vi "Autonomous Independent.vi"   [LabVIEW 2017]
doc: "This VI is called when autonomous begins, and will automatically be terminated when autonomous ends. You can carry out timed or sensor driven robot movement independently without needing to return to the caller."
uses:
  <vilib>/Rock Robotics/WPI/Utilities/WPI_GetSetVariantRefNum.vi
  <vilib>/Rock Robotics/Network Tables/NT Read String.vi
  <vilib>/Rock Robotics/Network Tables/NT Write Numeric Array.vi
  <vilib>/Rock Robotics/Network Tables/NT Read Number.vi
  <vilib>/Rock Robotics/Network Tables/NT Read Boolean.vi
panel:
  # "Be sure to right-click and choose Data Operations>>Make Current Value default if you want to save the array values with the VI"
types:
  T1 = typedef "WPI_JoystickDevRef.ctl" = cluster{"Device":T2}
  T2 = typedef "WPI_JoystickDeviceEnum.ctl" = enum16{"USB 0", "USB 1", "USB 2", "USB 3", "USB 4", "USB 5"}
  T3 = typedef "WPI_RobotDriveDevRef.ctl" = cluster{"DevStatus":errorcluster, "Motors[]":T4[], "Square Inputs":bool, "Max Output":dbl}
  T4 = typedef "WPI_MotorControlDeviceRef.ctl" = cluster{"DeviceStatus":errorcluster, "Type":T5, "PWM":cluster{"PWM Channel":T6, "DeadBand":T7}, "CAN":cluster{"Device Number":u8, "SetOutput VI Ref":variant, "GetOutput VI Ref":variant, "Enable VI Ref":variant, "Disable VI Ref":variant, "Data":variant}, "Invert":bool, "DIO PWM":cluster{"PWM \"Enable\" Channel":T6, "DIOChannel":T8, "PWM Rate":dbl}}
  T5 = typedef "WPI_MotorControlType.ctl" = enum16{"PWM", "CAN", "DIO PWM"}
  T6 = typedef "FPGA_DIOPWMChannel.ctl" = enum8{"PWM 0", "PWM 1", "PWM 2", "PWM 3", "PWM 4", "PWM 5", "PWM 6", "PWM 7", "PWM 8", "PWM 9", "PWM MXP 0", "PWM MXP 1", "PWM MXP 2", "PWM MXP 3", "PWM MXP 4", "PWM MXP 5", "PWM MXP 6", "PWM MXP 7", "PWM MXP 8", "PWM MXP 9", "Invalid"}
  T7 = typedef "WPI_PWMDeadband.ctl" = cluster{"Name":string, "maxPositivePwm":i32, "minPositivePwm":i32, "centerPwm":i32, "maxNegativePwm":i32, "minNegativePwm":i32, "angularRange":u16}
  T8 = typedef "FPGA_DIOChannel.ctl" = enum8{"DIO 0", "DIO 1", "DIO 2", "DIO 3", "DIO 4", "DIO 5", "DIO 6", "DIO 7", "DIO 8", "DIO 9", "DIO MXP 0", "DIO MXP 1", "DIO MXP 2", "DIO MXP 3", "DIO MXP 4", "DIO MXP 5", "DIO MXP 6", "DIO MXP 7", "DIO MXP 8", "DIO MXP 9", "DIO MXP 10", "DIO MXP 11", "DIO MXP 12", "DIO MXP 13", "DIO MXP 14", "DIO MXP 15", "SPI Port CS1", "SPI Port CS2", "SPI Port CS3", "SPI Port MISO", "SPI Port MOSI", "Invalid"}
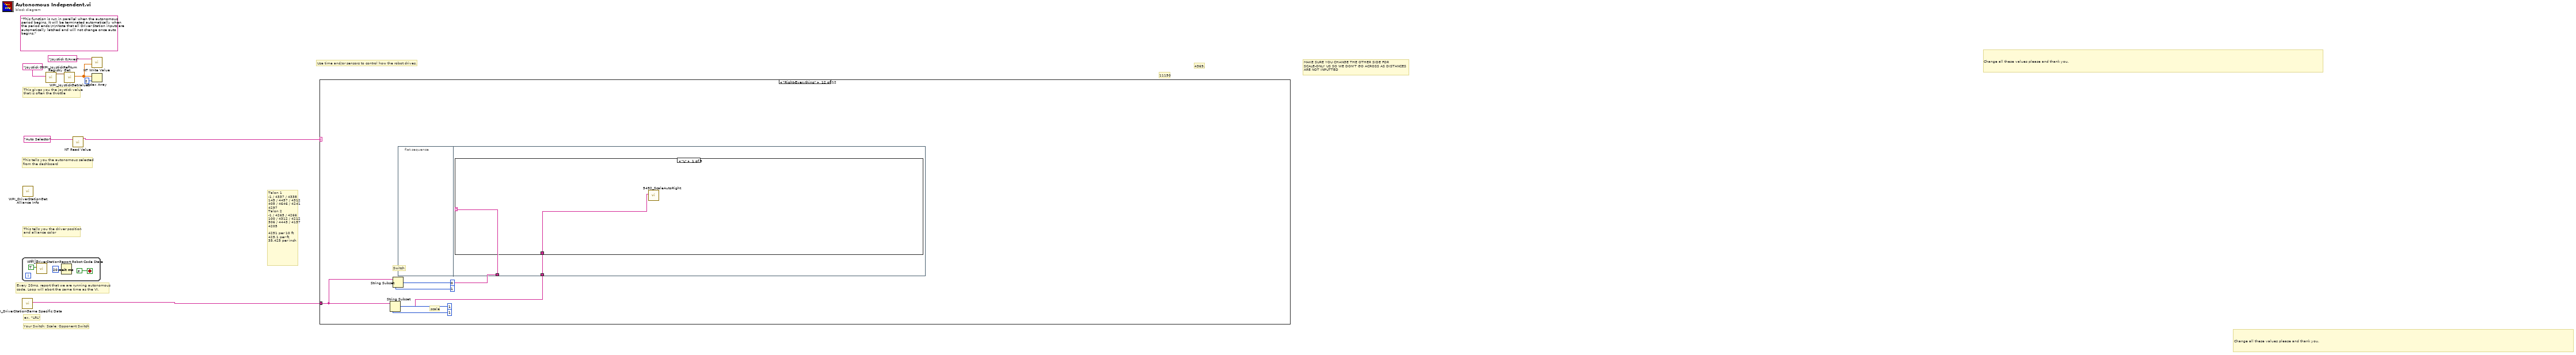
[diagram p0: block diagram]
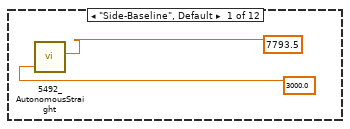
[diagram p2: hidden frame]
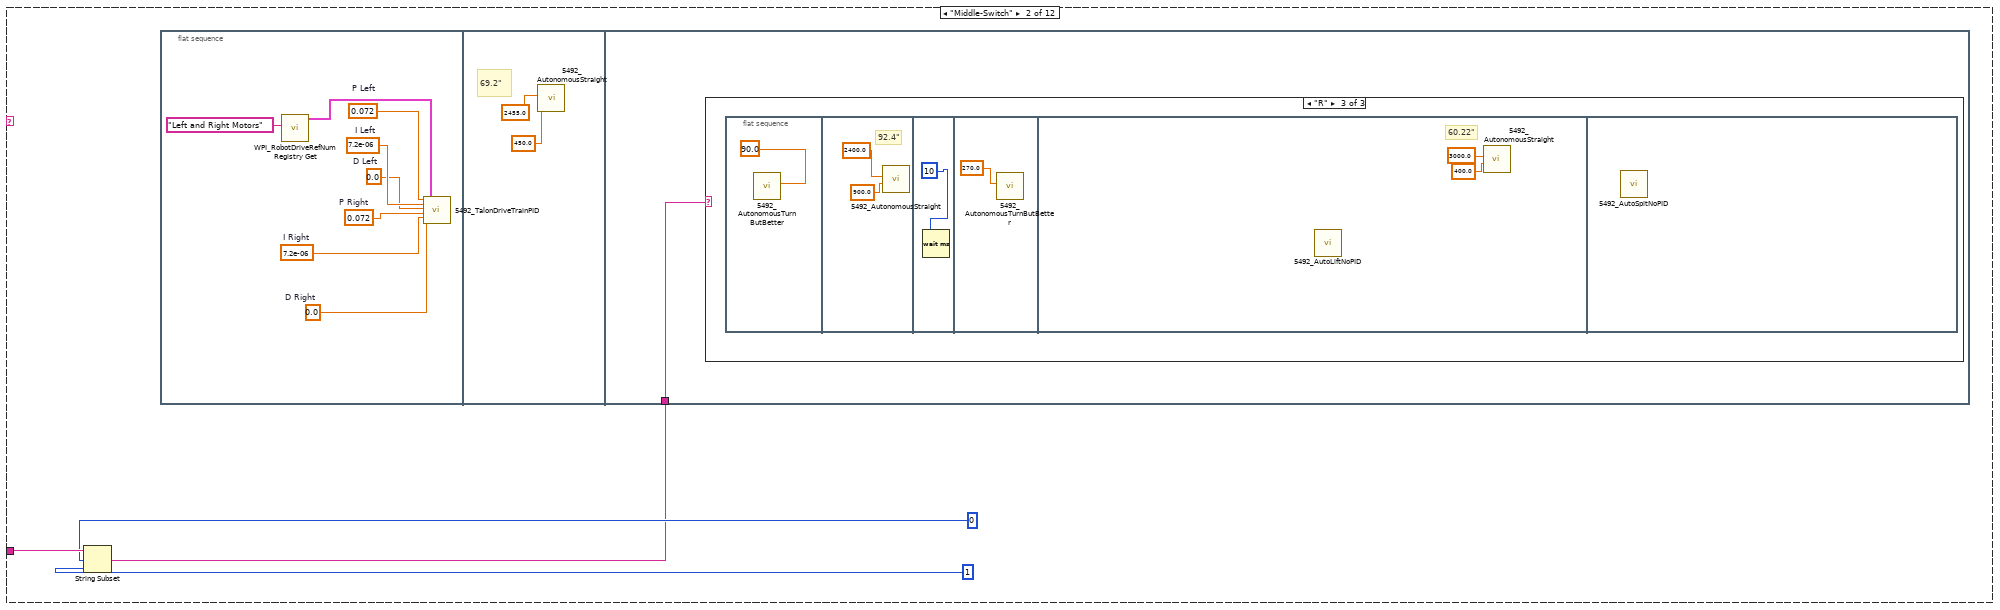
[diagram p3: hidden frame]
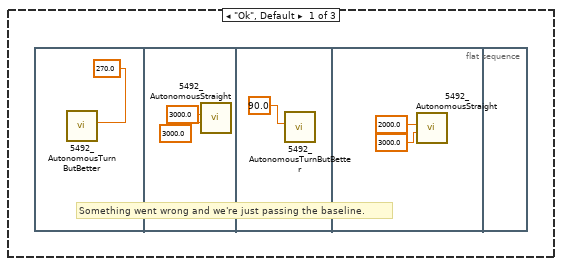
[diagram p4: hidden frame]
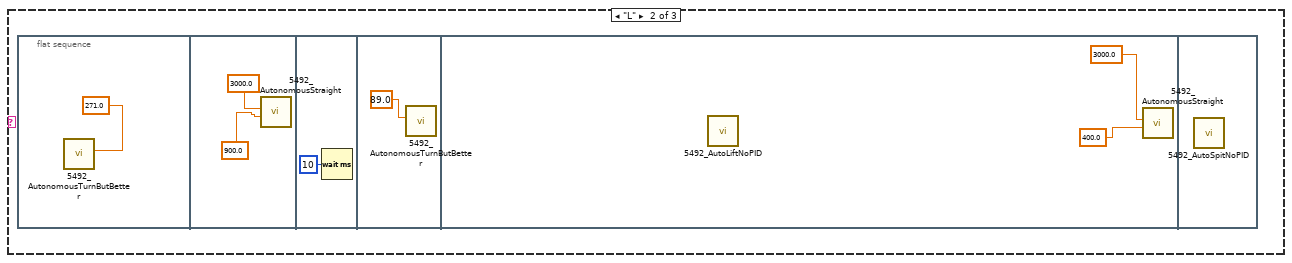
[diagram p5: hidden frame]
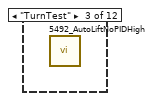
[diagram p6: hidden frame]
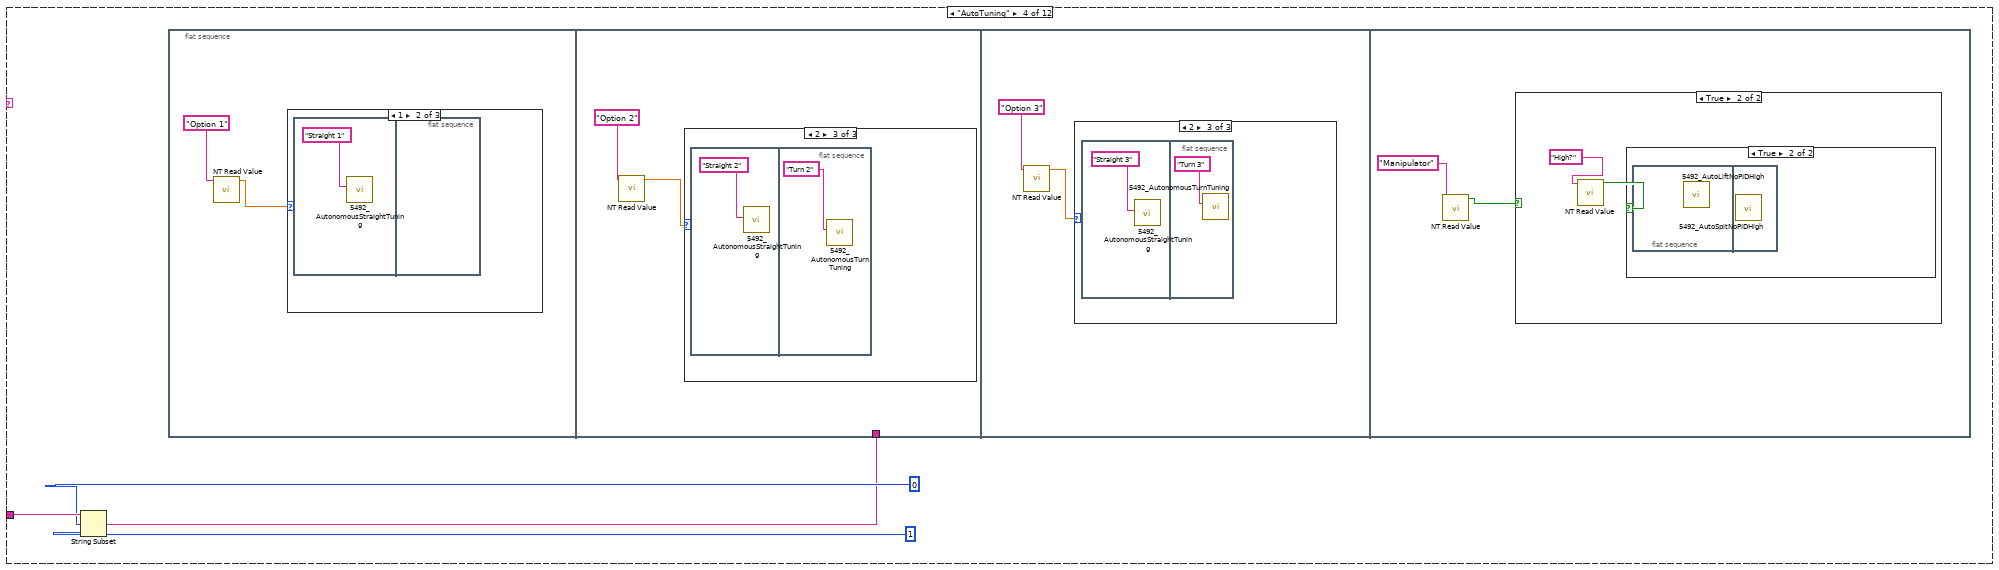
[diagram p7: hidden frame]
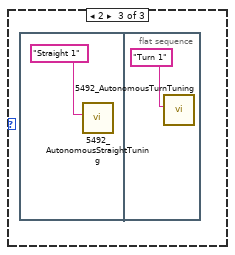
[diagram p9: hidden frame]
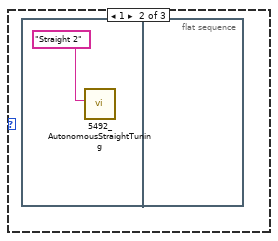
[diagram p11: hidden frame]
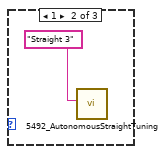
[diagram p13: hidden frame]
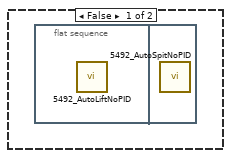
[diagram p15: hidden frame]
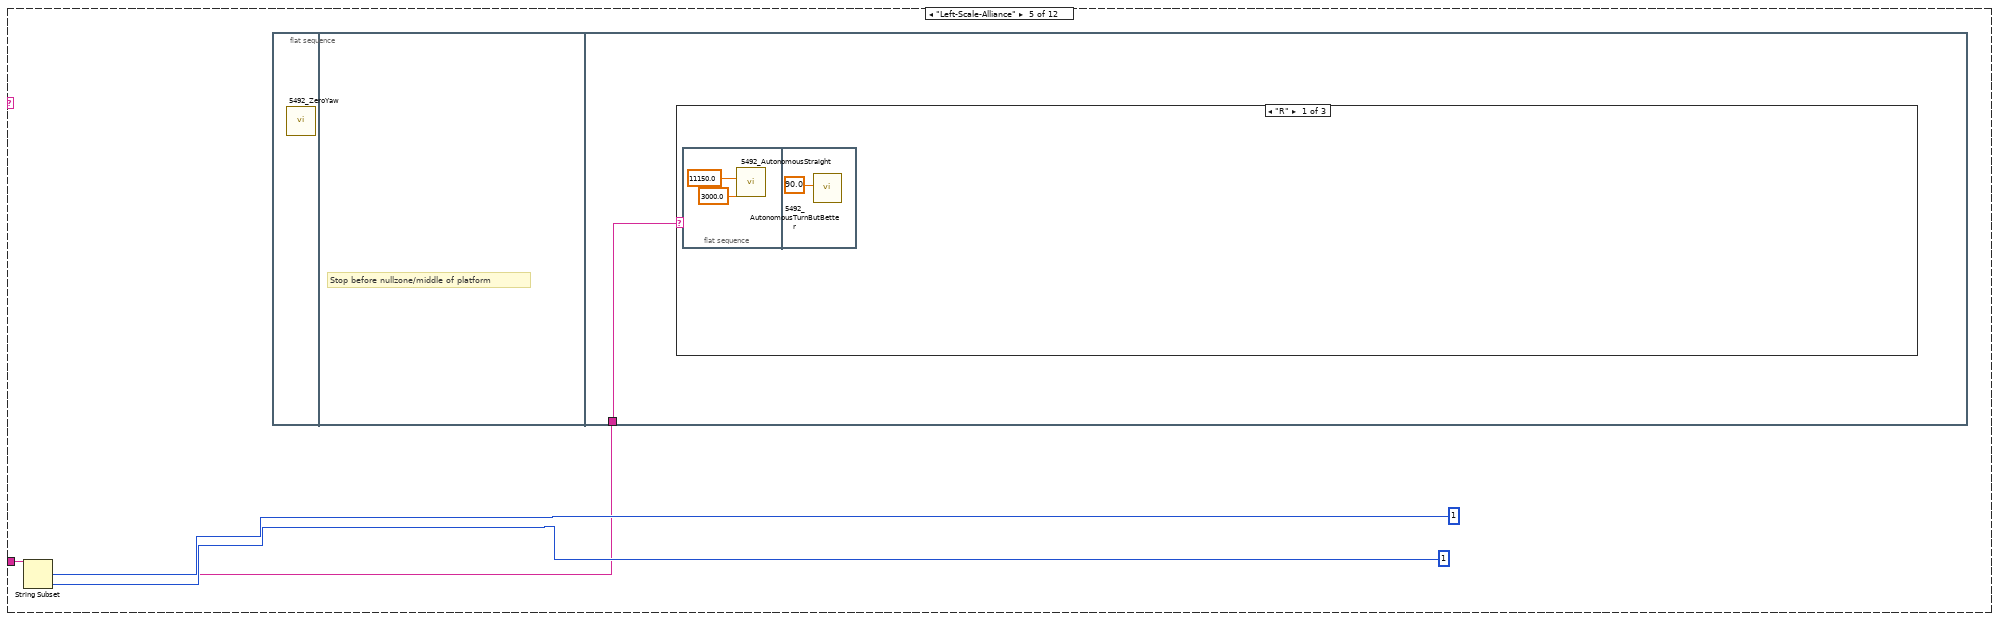
[diagram p16: hidden frame]
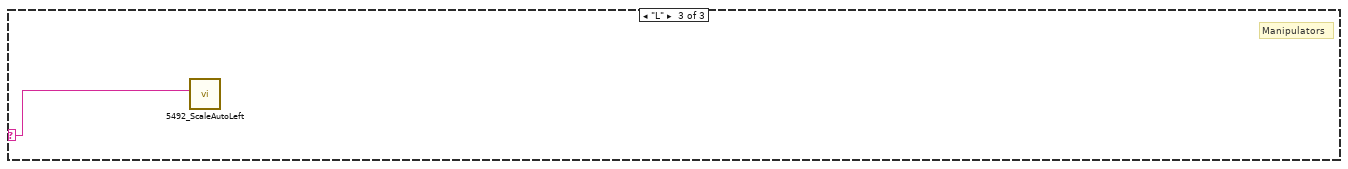
[diagram p18: hidden frame]
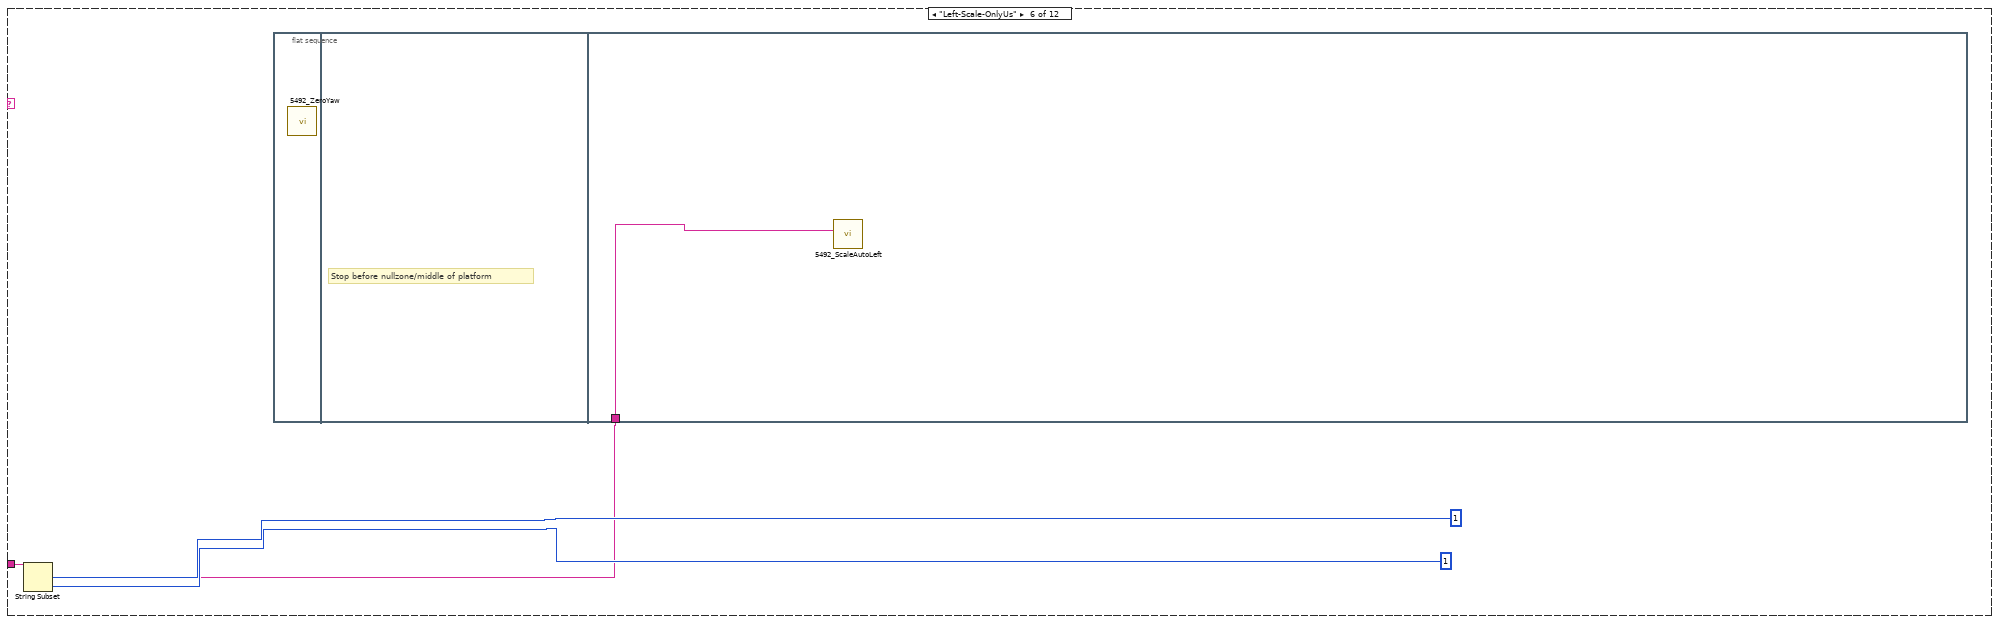
[diagram p19: hidden frame]
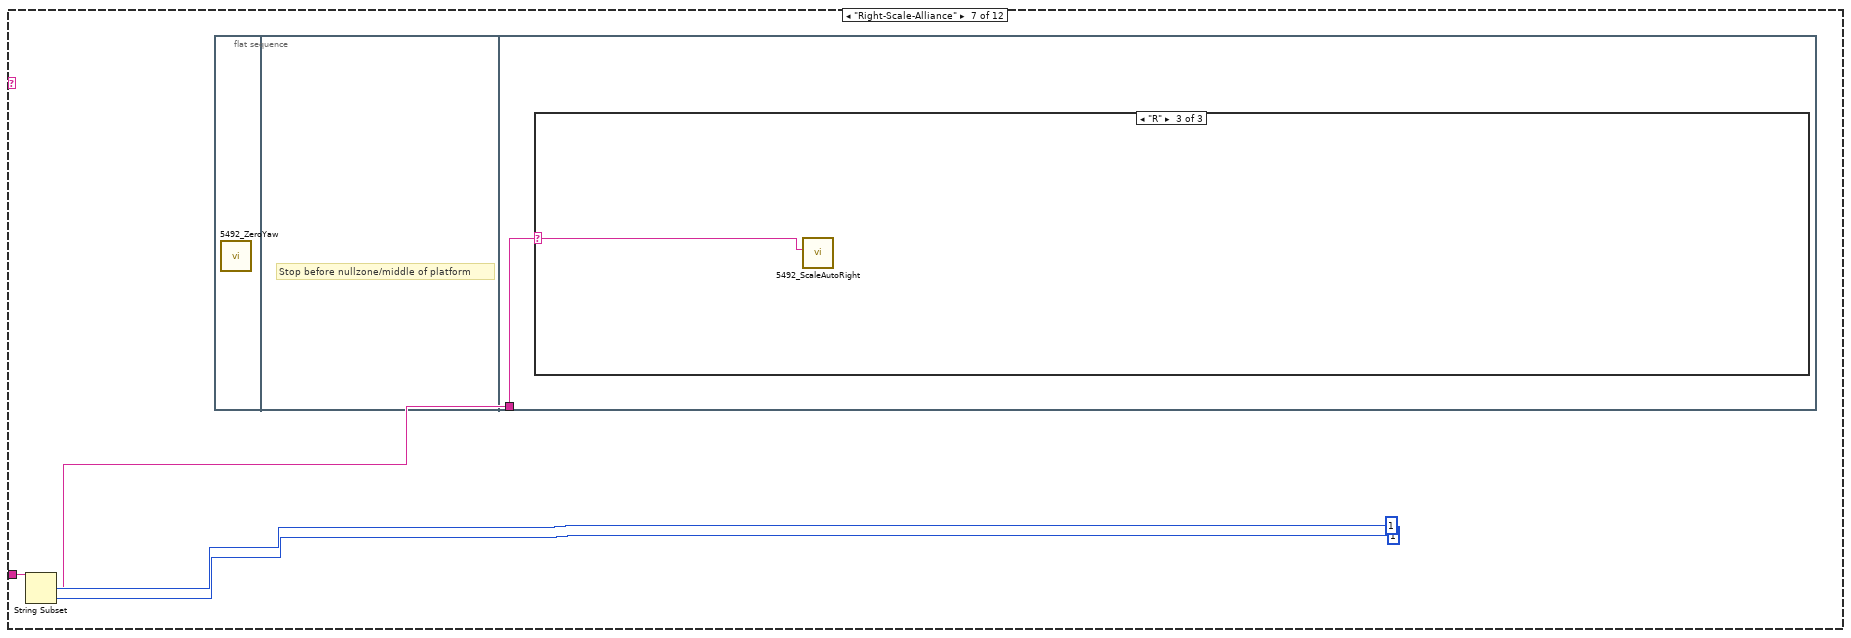
[diagram p20: hidden frame]
diagram:
  (unwired) "This function is run in parallel when the autonomous period begins. It will be terminated automatically when the period ends.\n\nNote that all Driver Station inputs are automatically latched and will not change once auto begins."
  # "4369."
  # "11150"
  # "MAKE SURE YOU CHANGE THE OTHER SIDE FOR\nSCALE-ONLY US SO WE DON'T GO ACROSS AS DISTANCES\nARE NOT INPUTTED"
  # "Talon 1\n-1 / 4337 / 4338\n145 / 4457 / 4312\n405 / 4646 / 4241\n4297\nTalon 2\n-1 / 4265 / 4266\n100 / 4312 / 4212\n306 / 4443 / 4137\n4205\n\n4251 per 10 ft\n425.1 per ft\n35.425 per inch"
  # "Change all these values please and thank you."
  # "Change all these values please and thank you."
  # "Your Switch; Scale; Opponent Switch"
  # "ex. \"LRL\""
  # "This tells you the autonomous selected\nfrom the dashboard"
  # "Every 20ms, report that we are running autonomous\ncode. Loop will abort the same time as the VI."
  # "This gives you the joystick value\nthat is often the throttle"
  # "Use time and/or sensors to control how the robot drives."
  # "This tells you the driver position\nand alliance color"
  n1 = while {
    stop <- FALSE stop-if-true
    n2 = call <vilib>:"WPI_DriverStationReport Robot Code State.vi"("Autonomous"=TRUE) -> ()  [unwired: 10 in, 1 out]
    n3 = Wait (ms)(milliseconds to wait=u32 20) -> ()  [unwired: 1 out]
  }
  n4 = call <vilib>:"WPI_DriverStationGame Specific Data.vi"() -> ("Game Specific Data"=w1:string)  [unwired: 11 in]
  n5 = call <vilib>:"WPI_DriverStationGet Alliance Info.vi"() -> ()  [unwired: 12 out]
  n6 = call <vilib>:"WPI_JoystickRefNum Registry Get.vi"("refnum name"="Joystick 0") -> ("JoystickDevRef"=w7:T1)  [unwired: 1 in, 9 out]
  n7 = call <vilib>:"WPI_JoystickGetValues.vi"("JoystickDevRef"=w7) -> ("Axes"=w3:dbl[])  [unwired: 6 in, 4 out]
  n8 = call-poly <vilib>:"NT Read Value.vi"("Name"="Auto Selector") -> ("String"=w4:string)  [unwired: 9 in, 1 out]
  n9 = call-poly <vilib>:"NT Write Value.vi"("Numeric Array"=w3, "Name"="Joystick 0/Axes") -> ()  [unwired: 9 in, 1 out]
  n10 = Index Array(array=w3, index=2) -> ()  [unwired: 1 out]
  n11 = case shown="\"Right-Everything\"" w4 {
    tunnel: w1 -> [_ w17 _ w52 w75 w84 w89 w98 w101 w117 w138 w168]
    frame "Side-Baseline", Default {
      n12 = call "5492_AutonomousStraight.vi"("Length"=3000.0, "Position Goal"=7793.5) -> ()  [unwired: 9 in, 1 out]
    }
    frame "Middle-Switch" {
      n13 = String Subset(string=w17, offset (0)=0, length (rest)=1 ("length (rest)")) -> (substring=w14:string)
      n14 = flat-sequence {
        tunnel: w14 -> [w28]
        frame #0 {
          w20 = 0.0  # D Right
          w21 = 7.2e-06  # I Right
          w22 = 0.072  # P Right
          w23 = 0.0  # D Left
          w24 = 7.2e-06  # I Left
          w25 = 0.072  # P Left
          n15 = call <vilib>:"WPI_RobotDriveRefNum Registry Get.vi"("refnum name"="Left and Right Motors") -> ("RobotDriveDevRef"=w18:T3)  [unwired: 9 in, 1 out]
          n16 = call "5492_TalonDriveTrainPID.vi"("P Left"=w25, "I Left"=w24, "D Left"=w23, "P Right"=w22, "I Right"=w21, "D Right"=w20, "RobotDriveDevRef 2"=w18) -> ()  [unwired: 12 in, 1 out]
        }
        frame #1 {
          # "69.2\""
          n17 = call "5492_AutonomousStraight.vi"("Length"=450.0, "Position Goal"=2455.0) -> ()  [unwired: 9 in, 1 out]
        }
        frame #2 {
          n18 = case shown="\"R\"" w28 {
            frame "Ok", Default {
              # "Something went wrong and we're just passing the baseline."
              n19 = flat-sequence {
                frame #0 {
                  n20 = call "5492_AutonomousTurnButBetter.vi"("Yaw Goallll"=270.0) -> ()  [unwired: 10 in, 1 out]
                }
                frame #1 {
                  n21 = call "5492_AutonomousStraight.vi"("Length"=3000.0, "Position Goal"=3000.0) -> ()  [unwired: 9 in, 1 out]
                }
                frame #2 {
                  n22 = call "5492_AutonomousTurnButBetter.vi"("Yaw Goallll"=90.0) -> ()  [unwired: 10 in, 1 out]
                }
                frame #3 {
                  n23 = call "5492_AutonomousStraight.vi"("Length"=3000.0, "Position Goal"=2000.0) -> ()  [unwired: 9 in, 1 out]
                }
                frame #4 {
                }
              }
            }
            frame "L" {
              n24 = flat-sequence {
                frame #0 {
                  n25 = call "5492_AutonomousTurnButBetter.vi"("Yaw Goallll"=271.0) -> ()  [unwired: 10 in, 1 out]
                }
                frame #1 {
                  n26 = call "5492_AutonomousStraight.vi"("Length"=900.0, "Position Goal"=3000.0) -> ()  [unwired: 9 in, 1 out]
                }
                frame #2 {
                  n27 = Wait (ms)(milliseconds to wait=u32 10) -> ()  [unwired: 1 out]
                }
                frame #3 {
                  n28 = call "5492_AutonomousTurnButBetter.vi"("Yaw Goallll"=89.0) -> ()  [unwired: 10 in, 1 out]
                }
                frame #4 {
                  n29 = call "5492_AutoLiftNoPID.vi"() -> ()  [unwired: 12 in]
                  n30 = call "5492_AutonomousStraight.vi"("Length"=400.0, "Position Goal"=3000.0) -> ()  [unwired: 9 in, 1 out]
                }
                frame #5 {
                  n31 = call "5492_AutoSpitNoPID.vi"() -> ()  [unwired: 12 in]
                }
              }
            }
            frame "R" {
              n32 = flat-sequence {
                frame #0 {
                  n33 = call "5492_AutonomousTurnButBetter.vi"("Yaw Goallll"=90.0) -> ()  [unwired: 10 in, 1 out]
                }
                frame #1 {
                  # "92.4\""
                  n34 = call "5492_AutonomousStraight.vi"("Length"=900.0, "Position Goal"=2400.0) -> ()  [unwired: 9 in, 1 out]
                }
                frame #2 {
                  n35 = Wait (ms)(milliseconds to wait=u32 10) -> ()  [unwired: 1 out]
                }
                frame #3 {
                  n36 = call "5492_AutonomousTurnButBetter.vi"("Yaw Goallll"=270.0) -> ()  [unwired: 10 in, 1 out]
                }
                frame #4 {
                  # "60.22\""
                  n37 = call "5492_AutoLiftNoPID.vi"() -> ()  [unwired: 12 in]
                  n38 = call "5492_AutonomousStraight.vi"("Length"=400.0, "Position Goal"=3000.0) -> ()  [unwired: 9 in, 1 out]
                }
                frame #5 {
                  n39 = call "5492_AutoSpitNoPID.vi"() -> ()  [unwired: 12 in]
                }
              }
            }
          }
        }
      }
    }
    frame "TurnTest" {
      n40 = call "5492_AutoLiftNoPIDHigh.vi"() -> ()  [unwired: 12 in]
    }
    frame "AutoTuning" {
      n41 = String Subset(string=w52, offset (0)=0, length (rest)=1 ("length (rest)")) -> (substring=w49:string)
      n42 = flat-sequence {
        tunnel: w49 -> [_]
        frame #0 {
          n43 = call-poly <vilib>:"NT Read Value.vi"("Name"="Option 1") -> ("Numeric"=w53:dbl)  [unwired: 9 in, 1 out]
          n44 = case shown="1" w53 {
            frame 0, Default {
            }
            frame 1 {
              n45 = flat-sequence {
                frame #0 {
                  n46 = call "5492_AutonomousStraightTuning.vi"("Straight Type"="Straight 1") -> ()  [unwired: 10 in, 1 out]
                }
                frame #1 {
                }
              }
            }
            frame 2 {
              n47 = flat-sequence {
                frame #0 {
                  n48 = call "5492_AutonomousStraightTuning.vi"("Straight Type"="Straight 1") -> ()  [unwired: 10 in, 1 out]
                }
                frame #1 {
                  n49 = call "5492_AutonomousTurnTuning.vi"("Turn Type"="Turn 1") -> ()  [unwired: 10 in, 1 out]
                }
              }
            }
          }
        }
        frame #1 {
          n50 = call-poly <vilib>:"NT Read Value.vi"("Name"="Option 2") -> ("Numeric"=w58:dbl)  [unwired: 9 in, 1 out]
          n51 = case shown="2" w58 {
            frame 0, Default {
            }
            frame 1 {
              n52 = flat-sequence {
                frame #0 {
                  n53 = call "5492_AutonomousStraightTuning.vi"("Straight Type"="Straight 2") -> ()  [unwired: 10 in, 1 out]
                }
                frame #1 {
                }
              }
            }
            frame 2 {
              n54 = flat-sequence {
                frame #0 {
                  n55 = call "5492_AutonomousStraightTuning.vi"("Straight Type"="Straight 2") -> ()  [unwired: 10 in, 1 out]
                }
                frame #1 {
                  n56 = call "5492_AutonomousTurnTuning.vi"("Turn Type"="Turn 2") -> ()  [unwired: 10 in, 1 out]
                }
              }
            }
          }
        }
        frame #2 {
          n57 = call-poly <vilib>:"NT Read Value.vi"("Name"="Option 3") -> ("Numeric"=w63:dbl)  [unwired: 9 in, 1 out]
          n58 = case shown="2" w63 {
            frame 0, Default {
            }
            frame 1 {
              n59 = call "5492_AutonomousStraightTuning.vi"("Straight Type"="Straight 3") -> ()  [unwired: 10 in, 1 out]
            }
            frame 2 {
              n60 = flat-sequence {
                frame #0 {
                  n61 = call "5492_AutonomousStraightTuning.vi"("Straight Type"="Straight 3") -> ()  [unwired: 10 in, 1 out]
                }
                frame #1 {
                  n62 = call "5492_AutonomousTurnTuning.vi"("Turn Type"="Turn 3") -> ()  [unwired: 10 in, 1 out]
                }
              }
            }
          }
        }
        frame #3 {
          n63 = call-poly <vilib>:"NT Read Value.vi"("Name"="Manipulator") -> ("Boolean"=w69:bool)  [unwired: 9 in, 1 out]
          n64 = case shown="True" w69 {
            frame False {
            }
            frame True {
              n65 = call-poly <vilib>:"NT Read Value.vi"("Name"="High?") -> ("Boolean"=w70:bool)  [unwired: 9 in, 1 out]
              n66 = case shown="True" w70 {
                frame False {
                  n67 = flat-sequence {
                    frame #0 {
                      n68 = call "5492_AutoLiftNoPID.vi"() -> ()  [unwired: 12 in]
                    }
                    frame #1 {
                      n69 = call "5492_AutoSpitNoPID.vi"() -> ()  [unwired: 12 in]
                    }
                  }
                }
                frame True {
                  n70 = flat-sequence {
                    frame #0 {
                      n71 = call "5492_AutoLiftNoPIDHigh.vi"() -> ()  [unwired: 12 in]
                    }
                    frame #1 {
                      n72 = call "5492_AutoSpitNoPIDHigh.vi"() -> ()  [unwired: 12 in]
                    }
                  }
                }
              }
            }
          }
        }
      }
    }
    frame "Left-Scale-Alliance" {
      n73 = String Subset(string=w75, offset (0)=1, length (rest)=1 ("length (rest)")) -> (substring=w72:string)
      n74 = flat-sequence {
        tunnel: w72 -> [w76]
        frame #0 {
          n75 = call "5492_ZeroYaw.vi"() -> ()  [unwired: 11 in, 1 out]
        }
        frame #1 {
          # "Stop before nullzone/middle of platform"
        }
        frame #2 {
          n76 = case shown="\"R\"" w76 {
            selector: w76 -> [_ _ w80]
            frame "R" {
              n77 = flat-sequence {
                frame #0 {
                  n78 = call "5492_AutonomousStraight.vi"("Length"=3000.0, "Position Goal"=11150.0) -> ()  [unwired: 9 in, 1 out]
                }
                frame #1 {
                  n79 = call "5492_AutonomousTurnButBetter.vi"("Yaw Goallll"=90.0) -> ()  [unwired: 10 in, 1 out]
                }
              }
            }
            frame "What?", Default {
            }
            frame "L" {
              # "Manipulators"
              n80 = call "5492_ScaleAutoLeft.vi"("Side"=w80) -> ()  [unwired: 11 in]
            }
          }
        }
      }
    }
    frame "Left-Scale-OnlyUs" {
      n81 = String Subset(string=w84, offset (0)=1, length (rest)=1 ("length (rest)")) -> (substring=w81:string)
      n82 = flat-sequence {
        tunnel: w81 -> [w85]
        frame #0 {
          n83 = call "5492_ZeroYaw.vi"() -> ()  [unwired: 11 in, 1 out]
        }
        frame #1 {
          # "Stop before nullzone/middle of platform"
        }
        frame #2 {
          n84 = call "5492_ScaleAutoLeft.vi"("Side"=w85) -> ()  [unwired: 11 in]
        }
      }
    }
    frame "Right-Scale-Alliance" {
      n85 = String Subset(string=w89, offset (0)=1, length (rest)=1 ("length (rest)")) -> (substring=w86:string)
      n86 = flat-sequence {
        tunnel: w86 -> [w90]
        frame #0 {
          n87 = call "5492_ZeroYaw.vi"() -> ()  [unwired: 11 in, 1 out]
        }
        frame #1 {
          # "Stop before nullzone/middle of platform"
        }
        frame #2 {
          n88 = case shown="\"R\"" w90 {
            selector: w90 -> [_ _ w94]
            frame "L" {
              n89 = flat-sequence {
                frame #0 {
                  n90 = call "5492_AutonomousStraight.vi"("Length"=3000.0, "Position Goal"=11150.0) -> ()  [unwired: 9 in, 1 out]
                }
                frame #1 {
                  n91 = call "5492_AutonomousTurnButBetter.vi"("Yaw Goallll"=270.0) -> ()  [unwired: 10 in, 1 out]
                }
              }
            }
            frame "What?", Default {
            }
            frame "R" {
              n92 = call "5492_ScaleAutoRight.vi"("Side"=w94) -> ()  [unwired: 11 in]
            }
          }
        }
      }
    }
    frame "Right-Scale-OnlyUs" {
      n93 = String Subset(string=w98, offset (0)=1, length (rest)=1 ("length (rest)")) -> (substring=w95:string)
      n94 = flat-sequence {
        tunnel: w95 -> [w99]
        frame #0 {
          n95 = call "5492_ZeroYaw.vi"() -> ()  [unwired: 11 in, 1 out]
        }
        frame #1 {
          # "Stop before nullzone/middle of platform"
        }
        frame #2 {
          n96 = call "5492_ScaleAutoRight.vi"("Side"=w99) -> ()  [unwired: 11 in]
        }
      }
    }
    frame "Left-Switch" {
      n97 = String Subset(string=w101, offset (0)=0, length (rest)=1 ("length (rest)")) -> (substring=w100:string)
      n98 = flat-sequence {
        tunnel: w100 -> [w106]
        frame #0 {
          n99 = call "5492_AutonomousStraight.vi"("Length"=1350.0, "Position Goal"=7795.0) -> ()  [unwired: 9 in, 1 out]
        }
        frame #1 {
          n100 = case shown="\"L\"" w106 {
            frame "R" {
              n101 = disable-structure shown="Disabled" {
                frame Disabled {
                  n102 = flat-sequence {
                    frame #0 {
                      n103 = call "5492_AutonomousStraight.vi"("Position Goal"=2000.0) -> ()  [unwired: 10 in, 1 out]
                    }
                    frame #1 {
                      n104 = call "5492_AutonomousTurnButBetter.vi"("Yaw Goallll"=90.0) -> ()  [unwired: 10 in, 1 out]
                    }
                    frame #2 {
                      n105 = call "5492_AutonomousStraight.vi"("Position Goal"=6500.0) -> ()  [unwired: 10 in, 1 out]
                    }
                    frame #3 {
                      n106 = call "5492_AutoLiftNoPID.vi"() -> ()  [unwired: 12 in]
                      n107 = call "5492_AutonomousTurnButBetter.vi"("Yaw Goallll"=90.0) -> ()  [unwired: 10 in, 1 out]
                    }
                    frame #4 {
                      n108 = call "5492_AutonomousStraight.vi"("Length"=100.0, "Position Goal"=500.0) -> ()  [unwired: 9 in, 1 out]
                    }
                    frame #5 {
                      n109 = call "5492_AutoSpitNoPID.vi"() -> ()  [unwired: 12 in]
                    }
                  }
                }
                frame Enabled {
                }
              }
            }
            frame "Que", Default {
            }
            frame "L" {
              n110 = flat-sequence {
                frame #0 {
                  n111 = call "5492_AutonomousTurnButBetter.vi"("Yaw Goallll"=90.0) -> ()  [unwired: 10 in, 1 out]
                }
                frame #1 {
                  n112 = call "5492_AutoLiftNoPID.vi"() -> ()  [unwired: 12 in]
                }
                frame #2 {
                  n113 = call "5492_AutonomousStraight.vi"("Length"=150.0, "Position Goal"=1000.0) -> ()  [unwired: 9 in, 1 out]
                }
                frame #3 {
                  n114 = call "5492_AutoSpitNoPID.vi"() -> ()  [unwired: 12 in]
                }
              }
            }
          }
        }
      }
    }
    frame "Right-Switch" {
      n115 = String Subset(string=w117, offset (0)=0, length (rest)=1 ("length (rest)")) -> (substring=w116:string)
      n116 = flat-sequence {
        tunnel: w116 -> [w122]
        frame #0 {
          n117 = call "5492_AutonomousStraight.vi"("Length"=3000.0, "Position Goal"=7795.0) -> ()  [unwired: 9 in, 1 out]
        }
        frame #1 {
          n118 = case shown="\"L\"" w122 {
            frame "L" {
              n119 = disable-structure shown="Disabled" {
                frame Disabled {
                  n120 = flat-sequence {
                    frame #0 {
                      n121 = call "5492_AutonomousStraight.vi"("Position Goal"=2000.0) -> ()  [unwired: 10 in, 1 out]
                    }
                    frame #1 {
                      n122 = call "5492_AutonomousTurnButBetter.vi"("Yaw Goallll"=270.0) -> ()  [unwired: 10 in, 1 out]
                    }
                    frame #2 {
                      n123 = call "5492_AutonomousStraight.vi"("Position Goal"=6500.0) -> ()  [unwired: 10 in, 1 out]
                    }
                    frame #3 {
                      n124 = call "5492_AutoLiftNoPID.vi"() -> ()  [unwired: 12 in]
                      n125 = call "5492_AutonomousTurnButBetter.vi"("Yaw Goallll"=270.0) -> ()  [unwired: 10 in, 1 out]
                    }
                    frame #4 {
                      n126 = call "5492_AutonomousStraight.vi"("Length"=100.0, "Position Goal"=500.0) -> ()  [unwired: 9 in, 1 out]
                    }
                    frame #5 {
                      n127 = call "5492_AutoSpitNoPID.vi"() -> ()  [unwired: 12 in]
                    }
                  }
                }
                frame Enabled {
                }
              }
            }
            frame "como", Default {
            }
            frame "R" {
              n128 = flat-sequence {
                frame #0 {
                  n129 = call "5492_AutonomousTurnButBetter.vi"("Yaw Goallll"=270.0) -> ()  [unwired: 10 in, 1 out]
                }
                frame #1 {
                  n130 = call "5492_AutoLiftNoPID.vi"() -> ()  [unwired: 12 in]
                }
                frame #2 {
                  n131 = call "5492_AutonomousStraight.vi"("Length"=150.0, "Position Goal"=1000.0) -> ()  [unwired: 9 in, 1 out]
                }
                frame #3 {
                  n132 = call "5492_AutoSpitNoPID.vi"() -> ()  [unwired: 12 in]
                }
              }
            }
          }
        }
      }
    }
    frame "Left-Everything" {
      # "scale"
      # "Switch"
      n133 = String Subset(string=w138, offset (0)=1, length (rest)=1 ("length (rest)")) -> (substring=w132:string)
      n134 = String Subset(string=w138, offset (0)=0, length (rest)=1 ("length (rest)")) -> (substring=w133:string)
      n135 = flat-sequence {
        tunnel: w133 -> [w140]
        tunnel: w132 -> [w139]
        frame #0 {
        }
        frame #1 {
          n136 = case shown="\"L\"" w140 {
            tunnel: w139 -> [w141 _ _]
            frame "R" {
              # "Scale"
              n137 = call "5492_ScaleAutoLeft.vi"("Side"=w141) -> ()  [unwired: 11 in]
            }
            frame "Que", Default {
            }
            frame "L" {
              # "Switch"
              n138 = flat-sequence {
                frame #0 {
                  w144 = 0.0  # D Right
                  w145 = 1e-05  # I Right
                  w146 = 0.1  # P Right
                  w147 = 0.0  # D Left
                  w148 = 1e-05  # I Left
                  w149 = 0.1  # P Left
                  n139 = call <vilib>:"WPI_RobotDriveRefNum Registry Get.vi"("refnum name"="Left and Right Motors") -> ("RobotDriveDevRef"=w142:T3)  [unwired: 9 in, 1 out]
                  n140 = call "5492_TalonDriveTrainPID.vi"("P Left"=w149, "I Left"=w148, "D Left"=w147, "P Right"=w146, "I Right"=w145, "D Right"=w144, "RobotDriveDevRef 2"=w142) -> ()  [unwired: 12 in, 1 out]
                }
                frame #1 {
                  n141 = call "5492_AutonomousStraight.vi"("Length"=3000.0, "Position Goal"=11150.0) -> ()  [unwired: 9 in, 1 out]
                }
                frame #2 {
                  n142 = call "5492_AutonomousTurnButBetter.vi"("Yaw Goallll"=137.0) -> ()  [unwired: 10 in, 1 out]
                }
                frame #3 {
                  n143 = call "5492_AutoLiftNoPID.vi"() -> ()  [unwired: 12 in]
                  n144 = call "5492_AutonomousStraight.vi"("Length"=300.0, "Position Goal"=1000.0) -> ()  [unwired: 9 in, 1 out]
                }
                frame #4 {
                }
                frame #5 {
                  n145 = call "5492_AutoSpitNoPID.vi"() -> ()  [unwired: 12 in]
                }
                frame #6 {
                  n146 = disable-structure shown="Disabled" {
                    frame Disabled {
                      n147 = call "5492_AutoDropNoPID.vi"() -> ()  [unwired: 12 in]
                    }
                    frame Enabled {
                    }
                  }
                  n148 = call "5492_AutonomousStraight.vi"("Length"=200.0, "Position Goal"=-500.0) -> ()  [unwired: 9 in, 1 out]
                }
                frame #7 {
                  n149 = call "5492_AutonomousStraight.vi"("Length"=200.0, "Position Goal"=500.0) -> ()  [unwired: 9 in, 1 out]
                }
                frame #8 {
                  n150 = call "5492_AutoGrab.vi"() -> ()  [unwired: 12 in]
                }
                frame #9 {
                  n151 = call "5492_AutonomousTurnButBetter.vi"("Yaw Goallll"=223.0) -> ()  [unwired: 10 in, 1 out]
                }
                frame #10 {
                  n152 = call "5492_AutoLiftNoPID.vi"() -> ()  [unwired: 12 in]
                  n153 = call "5492_AutonomousStraight.vi"("Length"=300.0, "Position Goal"=2500.0) -> ()  [unwired: 9 in, 1 out]
                }
                frame #11 {
                  n154 = call "5492_AutoSpitNoPID.vi"() -> ()  [unwired: 12 in]
                }
              }
            }
          }
        }
      }
    }
    frame "Right-Everything" {
      # "scale"
      # "Switch"
      n155 = String Subset(string=w168, offset (0)=1, length (rest)=1 ("length (rest)")) -> (substring=w162:string)
      n156 = String Subset(string=w168, offset (0)=0, length (rest)=1 ("length (rest)")) -> (substring=w163:string)
      n157 = flat-sequence {
        tunnel: w163 -> [w170]
        tunnel: w162 -> [w169]
        frame #0 {
        }
        frame #1 {
          n158 = case shown="\"L\"" w170 {
            tunnel: w169 -> [w171 _ _]
            frame "L" {
              n159 = call "5492_ScaleAutoRight.vi"("Side"=w171) -> ()  [unwired: 11 in]
            }
            frame "Que", Default {
            }
            frame "R" {
              n160 = flat-sequence {
                frame #0 {
                  w175 = 0.0  # D Right
                  w172 = 1e-05  # I Right
                  w176 = 0.1  # P Right
                  w177 = 0.0  # D Left
                  w178 = 1e-05  # I Left
                  w179 = 0.1  # P Left
                  n161 = call <vilib>:"WPI_RobotDriveRefNum Registry Get.vi"("refnum name"="Left and Right Motors") -> ("RobotDriveDevRef"=w173:T3)  [unwired: 9 in, 1 out]
                  n162 = call "5492_TalonDriveTrainPID.vi"("P Left"=w179, "I Left"=w178, "D Left"=w177, "P Right"=w176, "I Right"=w172, "D Right"=w175, "RobotDriveDevRef 2"=w173) -> ()  [unwired: 12 in, 1 out]
                }
                frame #1 {
                  n163 = call "5492_AutonomousStraight.vi"("Length"=3000.0, "Position Goal"=11150.0) -> ()  [unwired: 9 in, 1 out]
                }
                frame #2 {
                  n164 = call "5492_AutonomousTurnButBetter.vi"("Yaw Goallll"=223.0) -> ()  [unwired: 10 in, 1 out]
                }
                frame #3 {
                  n165 = call "5492_AutoLiftNoPID.vi"() -> ()  [unwired: 12 in]
                  n166 = call "5492_AutonomousStraight.vi"("Length"=300.0, "Position Goal"=1000.0) -> ()  [unwired: 9 in, 1 out]
                }
                frame #4 {
                }
                frame #5 {
                  n167 = call "5492_AutoSpitNoPID.vi"() -> ()  [unwired: 12 in]
                }
                frame #6 {
                  n168 = disable-structure shown="Disabled" {
                    frame Disabled {
                      n169 = call "5492_AutoDropNoPID.vi"() -> ()  [unwired: 12 in]
                    }
                    frame Enabled {
                    }
                  }
                  n170 = call "5492_AutonomousStraight.vi"("Length"=200.0, "Position Goal"=-500.0) -> ()  [unwired: 9 in, 1 out]
                }
                frame #7 {
                  n171 = call "5492_AutonomousStraight.vi"("Length"=200.0, "Position Goal"=750.0) -> ()  [unwired: 9 in, 1 out]
                }
                frame #8 {
                  n172 = call "5492_AutoGrab.vi"() -> ()  [unwired: 12 in]
                }
                frame #9 {
                  n173 = call "5492_AutonomousTurnButBetter.vi"("Yaw Goallll"=137.0) -> ()  [unwired: 10 in, 1 out]
                }
                frame #10 {
                  n174 = call "5492_AutoLiftNoPID.vi"() -> ()  [unwired: 12 in]
                  n175 = call "5492_AutonomousStraight.vi"("Length"=300.0, "Position Goal"=2500.0) -> ()  [unwired: 9 in, 1 out]
                }
                frame #11 {
                  n176 = call "5492_AutoSpitNoPID.vi"() -> ()  [unwired: 12 in]
                }
              }
            }
          }
        }
      }
    }
  }
